vi "Email Worker (SubVI).vi"(10 "Message Cluster":T1, 11 "Send Email?":bool) -> ()   [LabVIEW 2019]
doc: "Assembles the components of the message cluster into a more human-friendly email body message. Passes this, a constructed subject line, and the distribution list the Send Email subvi"
uses:
  Globals and Definitions/System Message.ctl
  a5bfeb0e-6229-4f50-a4ef-3b1ccf936079.vi
  Globals and Definitions/Initialization Globals.vi
panel:
  out "Receipients":string[](array[string])
  out "Message Subject Line":string
  out "Message Body":string
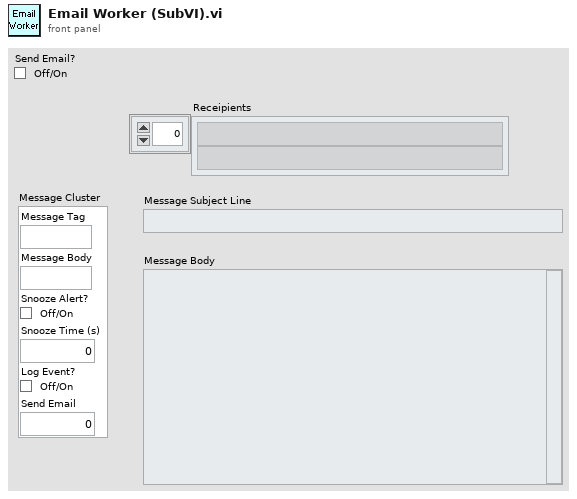
[diagram p1: front panel]
types:
  T1 = typedef "System Message.ctl" = cluster{"Message Tag":string, "Message Body":string, "Snooze Time (s)":dbl, "Snooze Alert?":bool, "Log Event?":bool, "Send Email":i32}
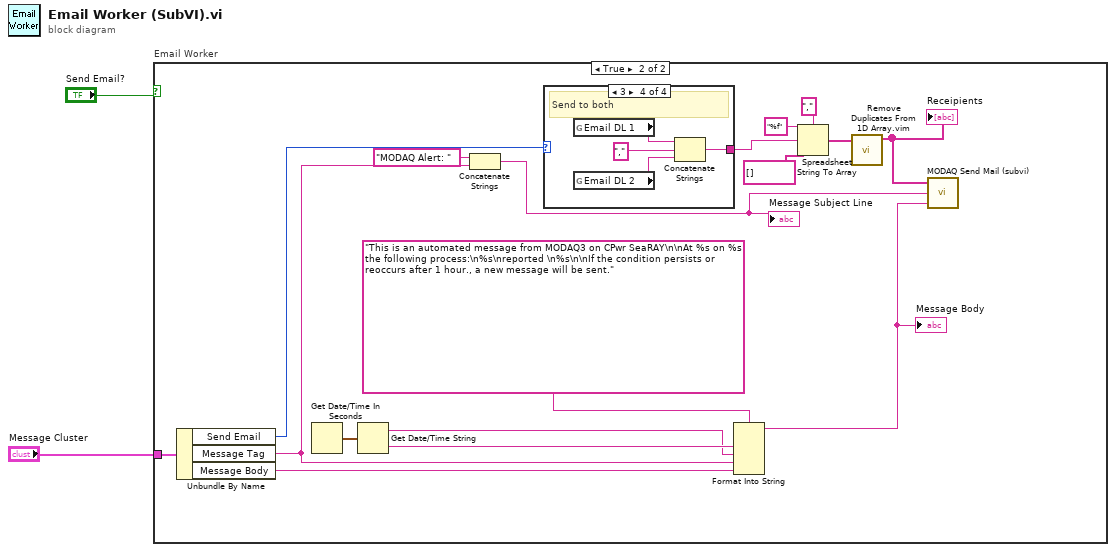
[diagram p0: block diagram]
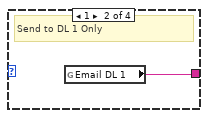
[diagram p4: hidden frame]
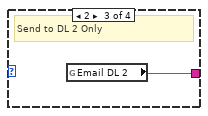
[diagram p5: hidden frame]
diagram:
  n1 = case "Email Worker" shown="True" "Send Email?" {
    tunnel: "Message Cluster" -> [_ w13]
    frame False {
    }
    frame True {
      n2 = Unbundle By Name(w13) -> ("Send Email"=w12:i32, "Message Tag"=w5:string, "Message Body"=w4:string)
      n3 = Get Date/Time In Seconds() -> (seconds since 1Jan1904=w3:timestamp)
      n4 = Get Date/Time String(seconds (now)=w3) -> (date string=w6:string, time string=w7:string)  [unwired: 2 in]
      n5 = Concatenate Strings("MODAQ Alert: " ("string"), w5) -> (w14:string)
      "Message Subject Line" <- w14
      n6 = case shown="3" w12 {
        tunnel: [_ w20 w21 w22] -> w16
        frame 0, Default {
        }
        frame 1 {
          # "Send to DL 1 Only"
          n7 = global read "Initialization Globals.vi" "Email DL 1"() -> (w20:string)
        }
        frame 2 {
          # "Send to DL 2 Only"
          n8 = global read "Initialization Globals.vi" "Email DL 2"() -> (w21:string)
        }
        frame 3 {
          # "Send to both"
          n9 = global read "Initialization Globals.vi" "Email DL 1"() -> (w25:string)
          n10 = global read "Initialization Globals.vi" "Email DL 2"() -> (w23:string)
          n11 = Concatenate Strings(w25, "," ("string"), w23) -> (w22:string)
        }
      }
      n12 = Format Into String(format string="This is an automated message from MODAQ3 on CPwr SeaRAY\n\nAt %s on %s the following process:\n%s\nreported \n%s\n\nIf the condition persists or reoccurs after 1 hour., a new message will be sent." ("string"), w7, w6, w5, w4) -> (resulting string=w8:string)  [unwired: 2 in, 1 out]
      "Message Body" <- w8
      n13 = Spreadsheet String To Array(delimiter (Tab)=",", format string="%f", spreadsheet string=w16, array type (2D Dbl)=string[] []) -> (array=w11:string[])
      n14 = call "Remove Duplicates From 1D Array.vim"("array"=w11) -> ("array with duplicates removed"=w10:string[])  [unwired: 10 in]
      "Receipients" <- w10
      n15 = call "MODAQ Send Mail (subvi).vi"("Message"=w8, "Subject"=w14, "To"=w10) -> ()  [unwired: 1 out]
    }
  }
